vi "Read U64.vi"(8 "error in (no error)":errorcluster, 9 "Timeout (ms)":i32, 11 "CIFChannels in":refnum<class "CIFChannels.lvclass">) -> (0 "error out":errorcluster, 1 "timed out?":bool, 2 "Data":u64, 3 "CIFChannels out":refnum<class "CIFChannels.lvclass">)   [LabVIEW 2021, in "CIFChannels.lvclass"]
uses:
  CIFChannels.lvclass
  CIFChannels.lvclass/CIFChannels.ctl
  CIFUtilities/CIFClocks/Typedef/Errors.ctl
  CIFCore/Common/Utilities/Append Error Location.vi
  CIFCore/Common/CIFCoreCommon.lvlib
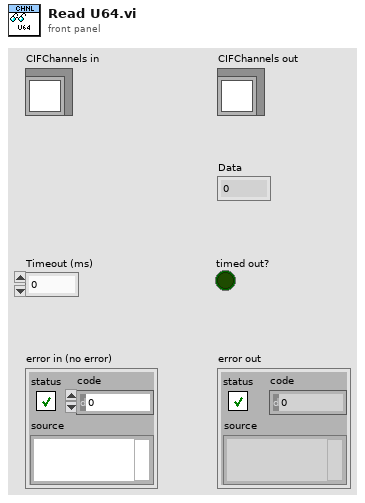
[diagram p1: front panel]
types:
  T1 = typedef "CIFCoreCommon.lvlib/Errors.ctl" = enum16{"Invalid Clock ID", "Long Sleep", "gRPC Server Not Found", "Config Parse", "Timestamp Wrap", "Delayed Execution", "Duplicate Channel", "Missing Channel", "Incorrect Type", "Flatten Error"}
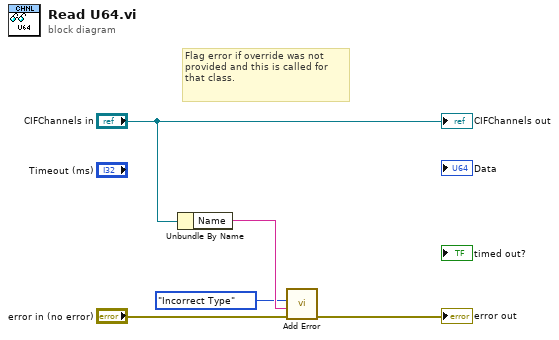
[diagram p0: block diagram]
diagram:
  # "Flag error if override was not provided and this is called for that class."
  n1 = Unbundle By Name("CIFChannels in") -> ("Name"=w3:string)
  n2 = call "Add Error.vi"("error in (no error)"="error in (no error)", "String to Append"=w3, "Error"=Errors."Incorrect Type") -> ("error out"=→"error out":errorcluster)  [unwired: 8 in]
  "CIFChannels out" <- "CIFChannels in"
